vi "VIRef_Updater.vi"(8 "error in (no error)":errorcluster, 11 "Numeric":dbl) -> (0 "error out":errorcluster, 2 "Is Strict?":bool, 3 "Class Name":string)   [LabVIEW 2020]
panel:
  out "Is Strict? 2":bool
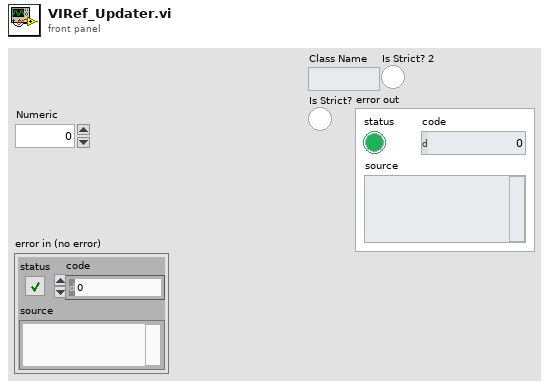
[diagram p1: front panel]
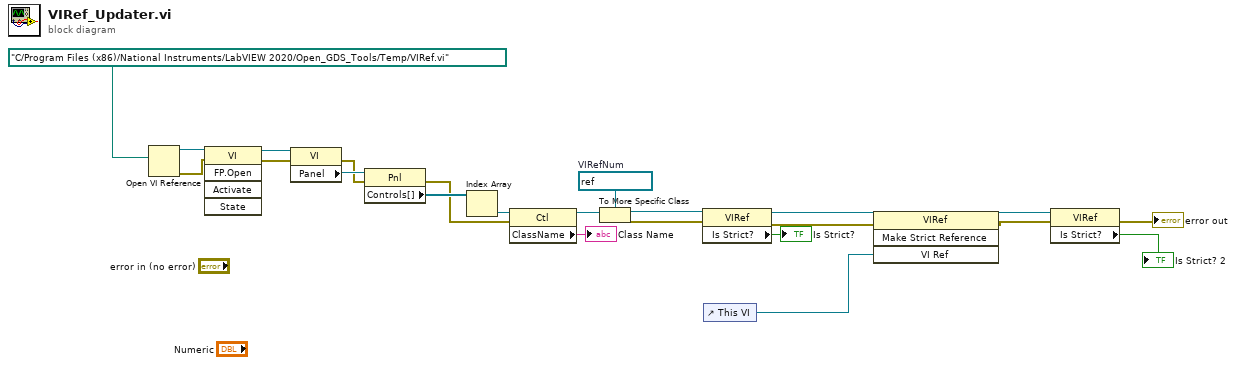
[diagram p0: block diagram]
diagram:
  w11 = refnum<vi> refnum  # VIRefNum
  n1 = Open VI Reference(vi path=path "C:/Program Files (x86)/National Instruments/LabVIEW 2020/Open_GDS_Tools/Temp/VIRef.vi") -> (vi reference=w22:refnum<vi>, error out=w21:errorcluster)  [unwired: 5 in]
  n2 = invoke class="VI" method="FP.Open"(reference=w22, error in=w21) -> (reference out=w20:refnum<vi>, error out=w19:errorcluster)  [unwired: 3 in, 3 out]
  n3 = property class="VI"(reference=w20, error in=w19) -> (error out=w17:errorcluster, "Panel"=w18:refnum<vi>)  [unwired: 1 out]
  n4 = property class="Pnl"(reference=w18, error in=w17) -> (error out=w14:errorcluster, "Controls[]"=w16:refnum<vi>[])  [unwired: 1 out]
  n5 = Index Array(array=w16) -> (element=w15:refnum<vi>)  [unwired: 1 in]
  n6 = property class="Ctl"(reference=w15, error in=w14) -> (reference out=w12:refnum<vi>, "ClassName"=→"Class Name":string)  [unwired: 1 out]
  n7 = To More Specific Class(target class=w11, reference=w12) -> (specific class reference=w10:refnum<vi>, error out=w9:errorcluster)  [unwired: 1 in]
  n8 = property class="VIRef"(reference=w10, error in=w9) -> (reference out=w7:refnum<vi>, error out=w3:errorcluster, "Is Strict?"=→"Is Strict?":bool)
  n9 = control-ref of="This VI"() -> (w6:refnum<vi>)
  n10 = invoke class="VIRef" method="Make Strict Reference"(reference=w7, error in=w3, "VI Ref"=w6) -> (reference out=w5:refnum<vi>, error out=w4:errorcluster)  [unwired: 1 in, 2 out]
  n11 = property class="VIRef"(reference=w5, error in=w4) -> (error out=→"error out":errorcluster, "Is Strict?"=→"Is Strict? 2":bool)  [unwired: 1 out]
